vi "19052 Get_DWLL_time.vi"(7 "Mode":T1, 8 "error in (no error)":errorcluster, 9 "Step":u16=1 min=1 max=99 step=1, 11 "VISA resource in":refnum<visa-resource-name>) -> (0 "error out":errorcluster, 1 "DWELL time":dbl format="%.1p", 2 "DWELL time string":string, 3 "VISA resource out":refnum<visa-resource-name>)   [LabVIEW 2015]
uses:
  Type Definitions/dc_ir_control.ctl
panel:
  out "output command":string
  # "Get DWLL time"
  # "[s]"
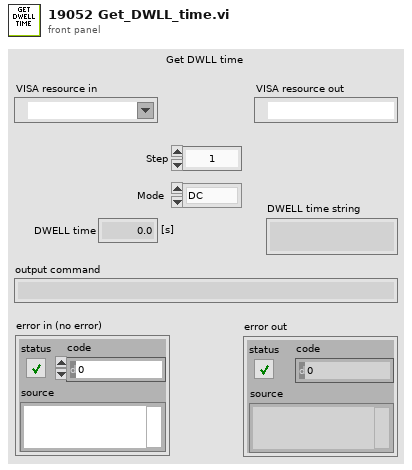
[diagram p1: front panel]
types:
  T1 = typedef "dc_ir_control.ctl" = enum16{"DC", "IR"}
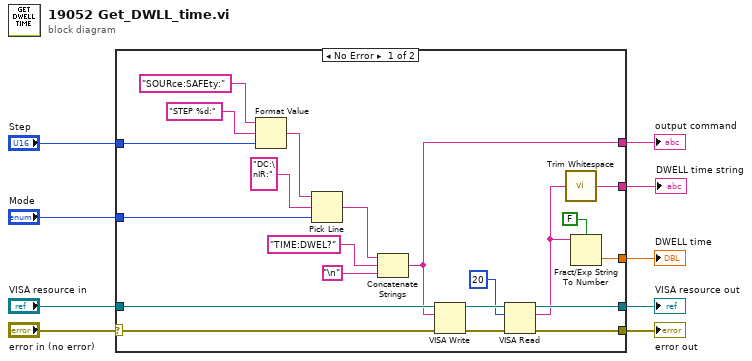
[diagram p0: block diagram]
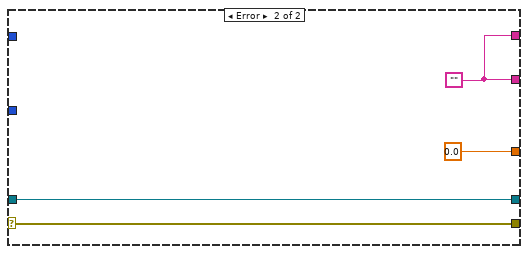
[diagram p2: hidden frame]
diagram:
  n1 = case shown="No Error" "error in (no error)" {
    selector: "error in (no error)" -> [w14 w33]
    tunnel: [w30 w33] -> w9
    tunnel: "VISA resource in" -> [w29 w34]
    tunnel: "Step" -> [w28 _]
    tunnel: [w19 w34] -> w7
    tunnel: [w16 w31] -> w6
    tunnel: "Mode" -> [w15 _]
    tunnel: [w13 0.0] -> w2
    tunnel: [w11 w31] -> w1
    frame No Error {
      n2 = Format Value(string ("")="SOURce:SAFEty:", format string="STEP %d:", value (0)=w28) -> (output string=w25:string)
      n3 = Pick Line(string ("")=w25, multi-line string="DC:\nIR:", line index=w15) -> (output string=w18:string)
      n4 = Concatenate Strings(w18, "TIME:DWEL?", "\n") -> (w16:string)
      n5 = VISA Write(VISA resource name=w29, write buffer=w16, error in (no error)=w14) -> (VISA resource name out=w21:refnum<visa-resource-name>, error out=w22:errorcluster)  [unwired: 1 out]
      n6 = VISA Read(VISA resource name=w21, byte count=u32 20, error in (no error)=w22) -> (VISA resource name out=w19:refnum<visa-resource-name>, read buffer=w10:string, error out=w30:errorcluster)  [unwired: 1 out]
      n7 = call <vilib>:"Trim Whitespace.vi"("string"=w10) -> ("trimmed string"=w11:string)  [unwired: 1 in]
      n8 = Fract/Exp String To Number(use system decimal point (T)=FALSE, string=w10) -> (number=w13:dbl)  [unwired: 2 in, 1 out]
    }
    frame Error {
      w31 = ""
    }
  }
  "error out" <- w9
  "VISA resource out" <- w7
  "output command" <- w6
  "DWELL time" <- w2
  "DWELL time string" <- w1
